vi "Set Initialization Data - RT Watchdog.vi"(8 "error in":errorcluster, 11 "cRIO NI 9205 Demo in":refnum<class "cRIO NI 9205 Demo.lvclass">) -> (0 "error out":errorcluster, 3 "cRIO NI 9205 Demo out":refnum<class "cRIO NI 9205 Demo.lvclass">)   [LabVIEW 2017, in "cRIO NI 9205 Demo.lvclass"]
doc: "In this VI you can set the initialization data of a statically-linked subWorker."
uses:
  cRIO NI 9205 Demo.lvclass
  RT Watchdog/Initialization Data.ctl
  RT Watchdog/Response Cases.ctl
  <vilib>/addons/_Workers/Library/Case Label.ctl
  <vilib>/RTwatchdog.llb/Watchdog expiration actions.ctl
  cRIO NI 9205 Demo.lvclass/cRIO NI 9205 Demo.ctl
  RT Watchdog/RT Watchdog.lvclass
  C:/Program Files (x86)/National Instruments/LabVIEW 2017/vi.lib/addons/_Workers/Library/Classes/Worker/Worker.lvclass
  <vilib>/addons/_Workers/Library/Workers.lvlib
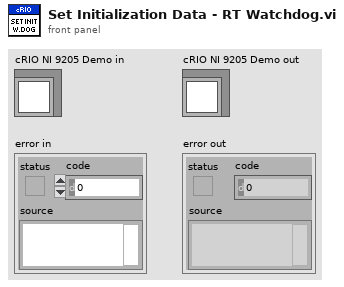
[diagram p1: front panel]
types:
  T1 = typedef "RT Watchdog.lvclass/Initialization Data.ctl" = cluster{"Response Cases":T2, "Debugging Mode?":bool, "expiration actions":T4, "timeout (1 sec)":dbl}
  T2 = typedef "RT Watchdog.lvclass/Response Cases.ctl" = cluster{"Watchdog Expired":T3}
  T3 = typedef "Workers.lvlib/Case Label.ctl" = string
  T4 = typedef "Watchdog expiration actions.ctl" = cluster{"reset system":bool, "restart LabVIEW Runtime":bool, "occurrence":bool, "trigger protocol":enum16{"active high", "active low", "open collector"}, "trigger line":enum16{"none", "line 0", "line 1", "line 2", "line 3", "line 4", "line 5", "line 6", "line 7", "SMB line 0"}, "disable watchdog on VI exit":bool}
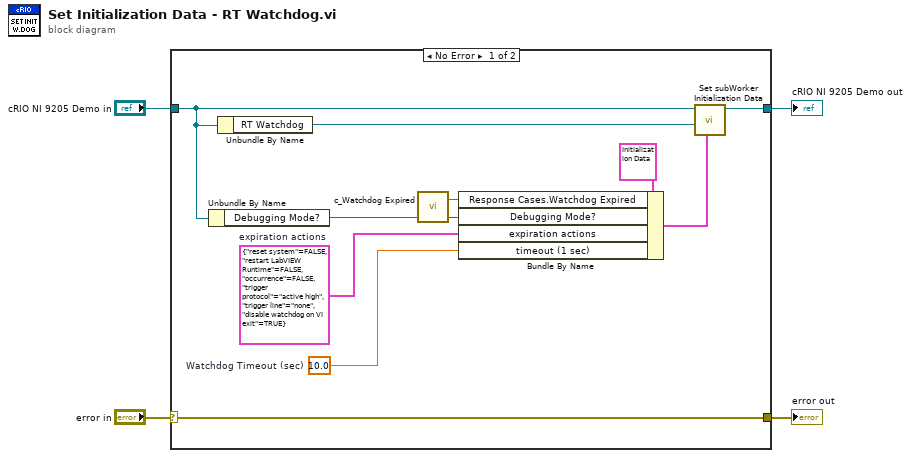
[diagram p0: block diagram]
diagram:
  n1 = case shown="No Error" "error in" {
    selector: "error in" -> [w14 w16]
    tunnel: [w14 w16] -> w3
    tunnel: [w12 w15] -> w2
    tunnel: "cRIO NI 9205 Demo in" -> [w9 w15]
    frame No Error {
      w7 = T4 {"reset system"=FALSE, "restart LabVIEW Runtime"=FALSE, "occurrence"=FALSE, "trigger protocol"=enum."active high", "trigger line"=enum."none", "disable watchdog on VI exit"=TRUE}  # expiration actions
      w6 = 10.0  # Watchdog Timeout (sec)
      n2 = Unbundle By Name(w9) -> ("Debugging Mode?"=w8:bool)
      n3 = Unbundle By Name(w9) -> ("RT Watchdog"=w13:refnum<class "RT Watchdog.lvclass">)
      n4 = call "c_Watchdog Expired.vi"() -> ("Case Label"=w5:T3)  [unwired: 1 in]
      n5 = Bundle By Name(cluster=T1 {"Response Cases"={"Watchdog Expired"=""}, "Debugging Mode?"=FALSE, "expiration actions"={"reset system"=FALSE, "restart LabVIEW Runtime"=FALSE, "occurrence"=FALSE, "trigger protocol"=enum."active high", "trigger line"=enum."none", "disable watchdog on VI exit"=TRUE}, "timeout (1 sec)"=1.0} ("Initialization Data"), "Response Cases.Watchdog Expired"=w5, "Debugging Mode?"=w8, "expiration actions"=w7, "timeout (1 sec)"=w6) -> (w10:T1)
      n6 = call-dynamic "Set subWorker Initialization Data.vi"("Initialization Data"=w10, "subWorker"=w13, "Worker"=w9) -> ("Worker out"=w12:refnum<class "cRIO NI 9205 Demo.lvclass">)  [unwired: 8 in]
    }
    frame Error {
    }
  }
  "error out" <- w3
  "cRIO NI 9205 Demo out" <- w2
